vi "Mes配置.vi"() -> (1 "MES[]":T1(array[cluster]), 3 "MES 配置 2":T2={"SITE"="A157", "OPERATION"="Z-TEST", "QTY"="1", "ACTIVITY"="", "RESOURCE"="A-6-Z-TEST", "NC_CODE"="Z-TEST_FAIL", "IP"="10.9.30.175", "PORT"="50100", "URL"="/manufacturing/IntegrationServlet?InterType=XML&message="})   [LabVIEW 2011]
uses:
  Button.ctl
panel:
  in  "MES 配置":T2={"SITE"="A157", "OPERATION"="Z-TEST", "QTY"="1", "ACTIVITY"="", "RESOURCE"="A-6-Z-TEST", "NC_CODE"="Z-TEST_FAIL", "IP"="10.9.30.175", "PORT"="50100", "URL"="/manufacturing/IntegrationServlet?InterType=XML&message="}
  in  "delete":T3
  in  "input":T3
  in  "新建":T3
  in  "Exit":T3
  in  "所有MES配置表":i32(listbox)
  in  "MES配置信息名称":string
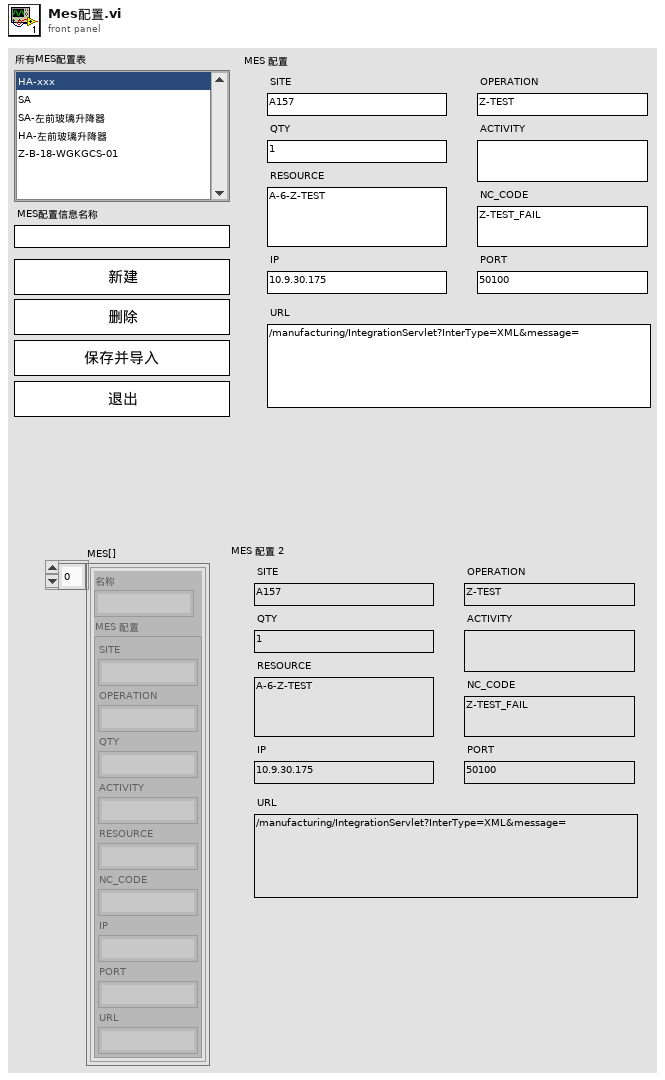
[diagram p1: front panel]
types:
  T1 = cluster{"名称":string, "MES 配置":cluster{"SITE":string, "OPERATION":string, "QTY":string, "ACTIVITY":string, "RESOURCE":string, "NC_CODE":string, "IP":string, "PORT":string, "URL":string}}[]
  T2 = cluster{"SITE":string, "OPERATION":string, "QTY":string, "ACTIVITY":string, "RESOURCE":string, "NC_CODE":string, "IP":string, "PORT":string, "URL":string}
  T3 = typedef "Button.ctl" = bool
  T4 = cluster{"名称":string, "电机位置":cluster{"左工位工作位置":cluster{"Axis":i16, "Distance":i32, "StrVel":i32, "MaxVel":i32}, "左工位抬起开关位置":cluster{"Axis":i16, "Distance":i32, "StrVel":i32, "MaxVel":i32}, "左工位按下开关位置":cluster{"Axis":i16, "Distance":i32, "StrVel":i32, "MaxVel":i32}, "右工位工作位置":cluster{"Axis":i16, "Distance":i32, "StrVel":i32, "MaxVel":i32}, "右工位抬起开关位置":cluster{"Axis":i16, "Distance":i32, "StrVel":i32, "MaxVel":i32}, "右工位按下开关位置":cluster{"Axis":i16, "Distance":i32, "StrVel":i32, "MaxVel":i32}}}
  T5 = cluster{"名称":string, "判定条件":cluster{"A1-A2电阻":cluster{"上限":dbl, "下限":dbl, "单位":string}, "A3-A4电阻":cluster{"上限":dbl, "下限":dbl, "单位":string}, "A4-A5电阻":cluster{"上限":dbl, "下限":dbl, "单位":string}, "A5-A6电阻":cluster{"上限":dbl, "下限":dbl, "单位":string}, "A1-A3电阻":cluster{"上限":dbl, "下限":dbl, "单位":string}, "A2-A6电阻":cluster{"上限":dbl, "下限":dbl, "单位":string}, "A1导地A3-A5电压":cluster{"上限":dbl, "下限":dbl, "单位":string}, "A2导地A6-A5电压":cluster{"上限":dbl, "下限":dbl, "单位":string}, "抬起开关A3-A5电压":cluster{"上限":dbl, "下限":dbl, "单位":string}, "按下开关A6-A5电压":cluster{"上限":dbl, "下限":dbl, "单位":string}, "背光电流":cluster{"上限":dbl, "下限":dbl, "单位":string}, "A1导地A6-A5电压":cluster{"上限":dbl, "下限":dbl, "单位":string}, "A2导地A3-A5电压":cluster{"上限":dbl, "下限":dbl, "单位":string}}}
  T6 = cluster{"名称":string, "MES 配置":cluster{"SITE":string, "OPERATION":string, "QTY":string, "ACTIVITY":string, "RESOURCE":string, "NC_CODE":string, "IP":string, "PORT":string, "URL":string}}
  T7 = enum16{"open", "replace", "create", "open or create", "replace or create", "replace or create with confirmation"}
  T8 = cluster{"SITE":string, "OPERATION":string, "QTY":string, "ACTIVITY":string, "RESOURCE":string, "NC_CODE":string, "IP":string, "PORT":string, "URL":string}[]
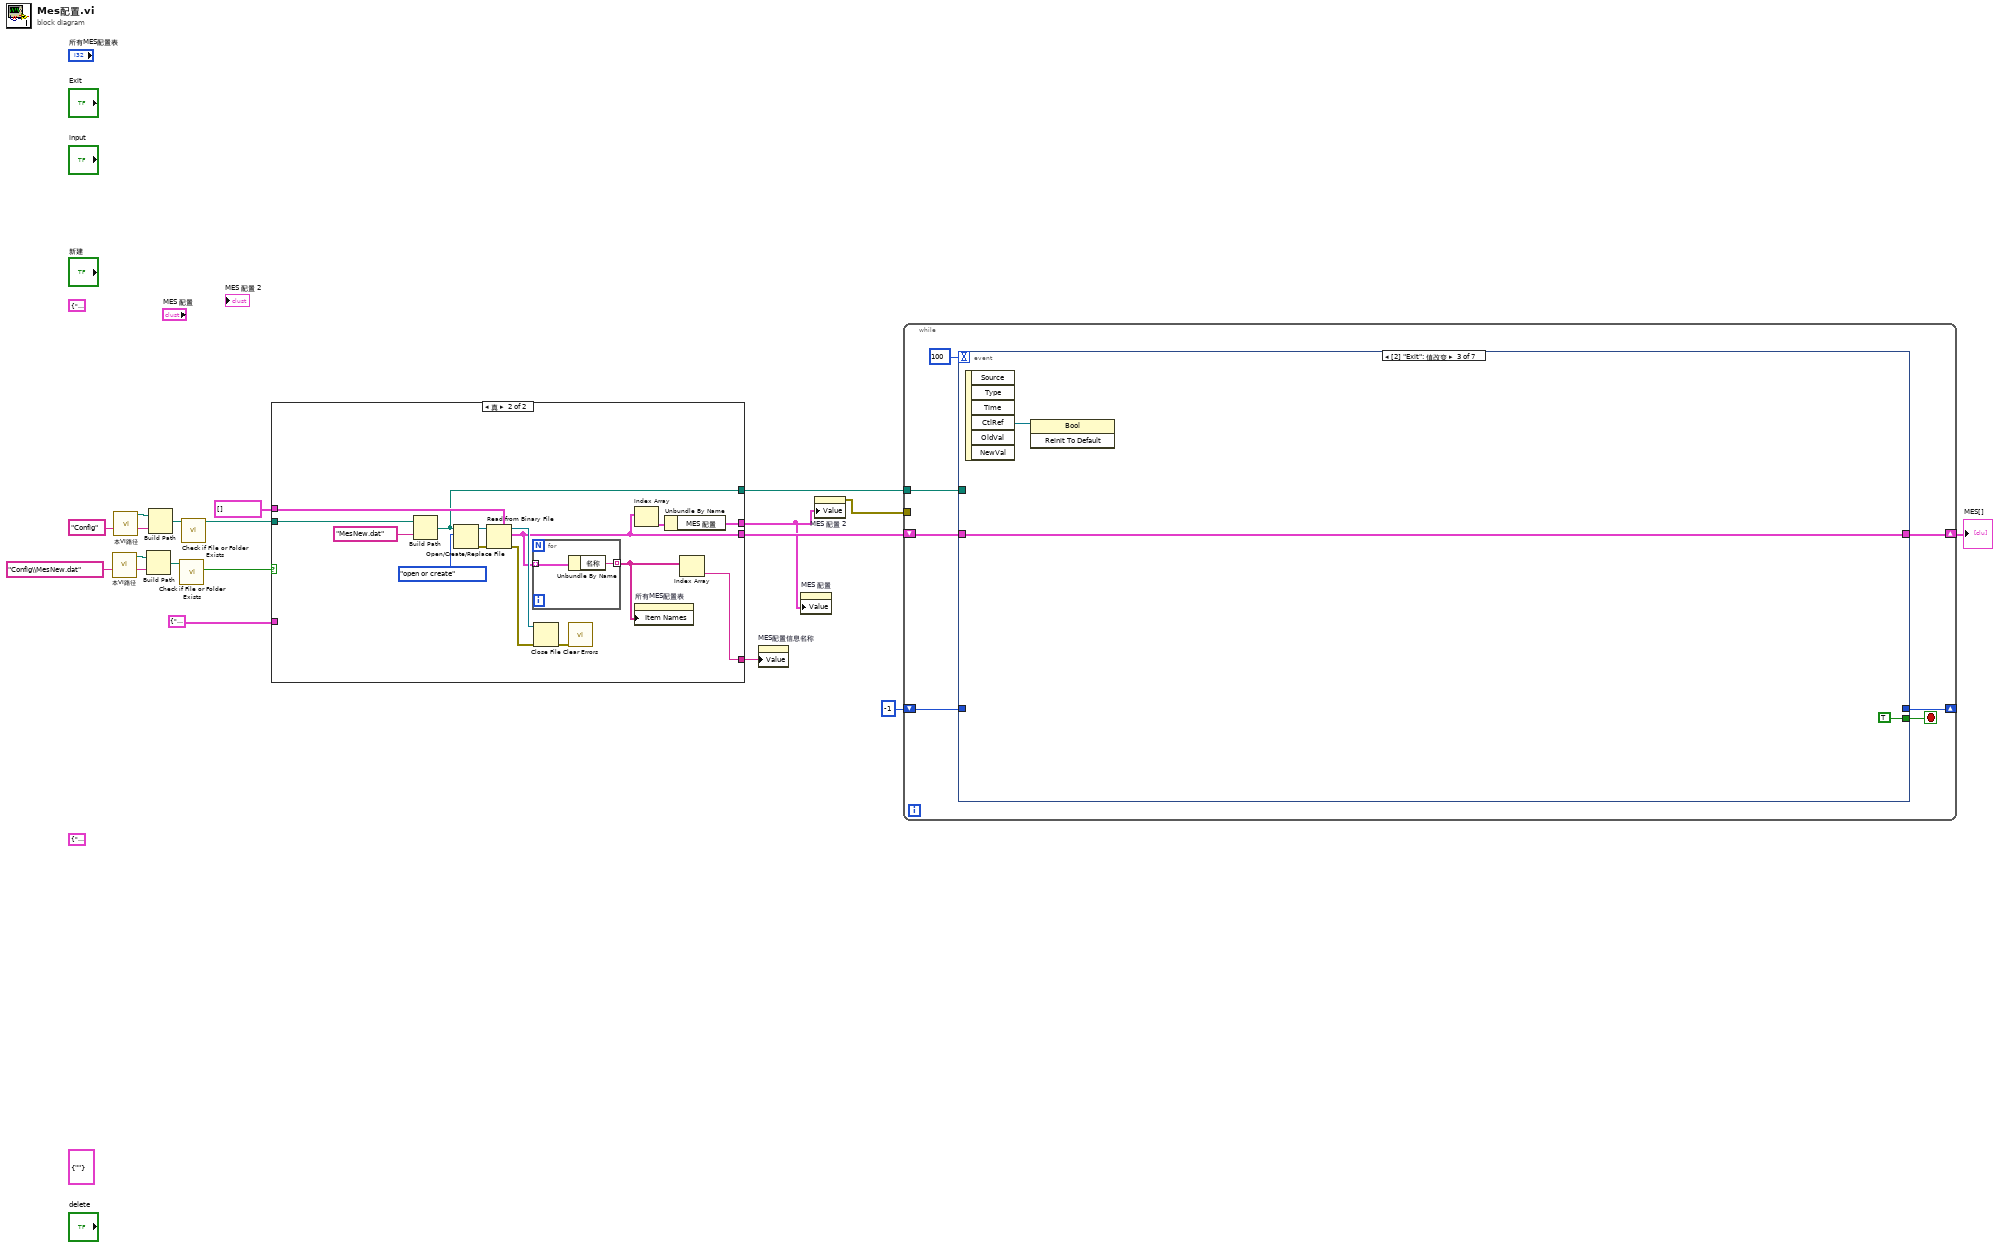
[diagram p0: block diagram]
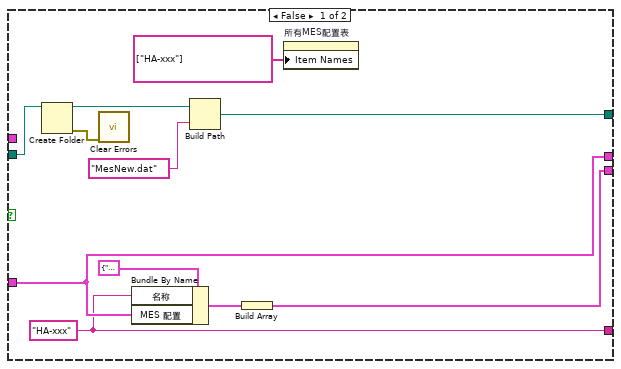
[diagram p2: hidden frame]
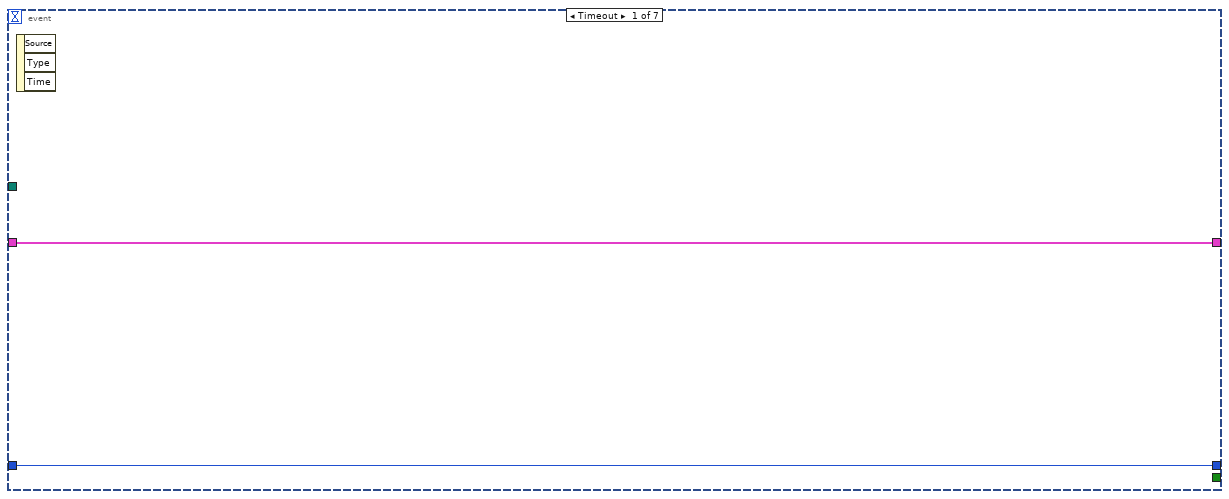
[diagram p3: hidden frame]
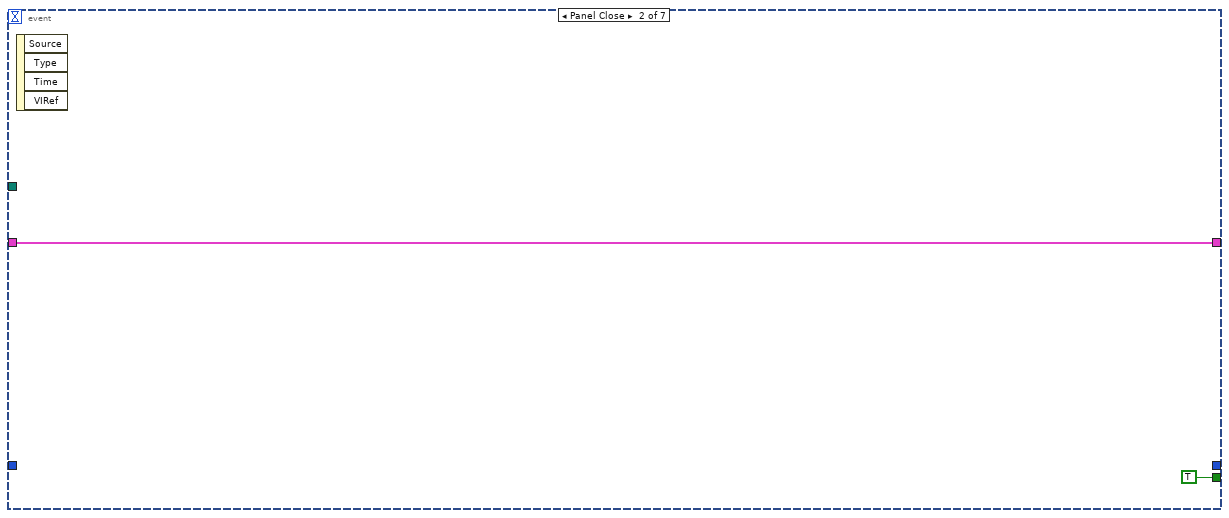
[diagram p4: hidden frame]
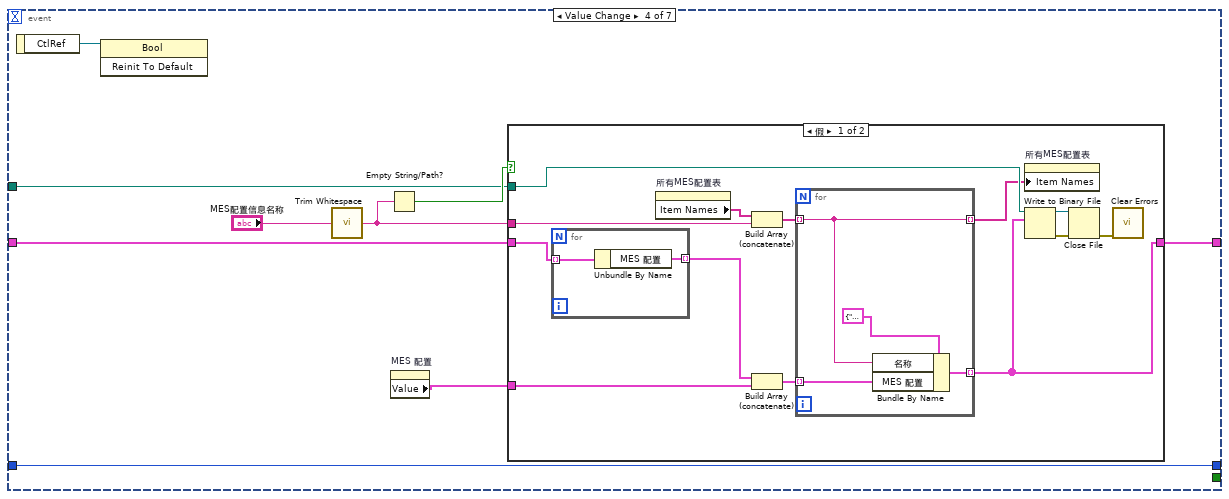
[diagram p5: hidden frame]
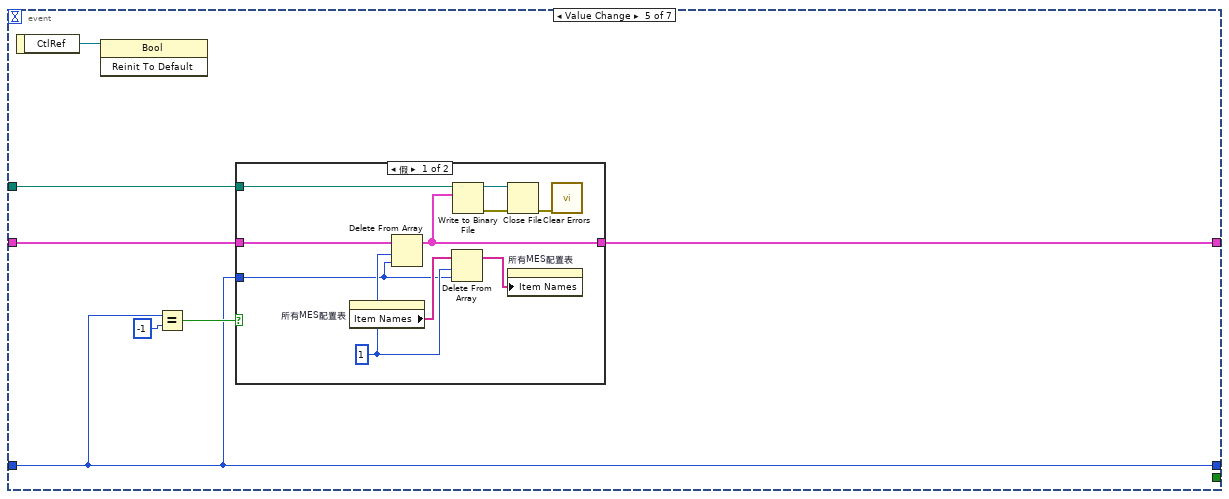
[diagram p7: hidden frame]
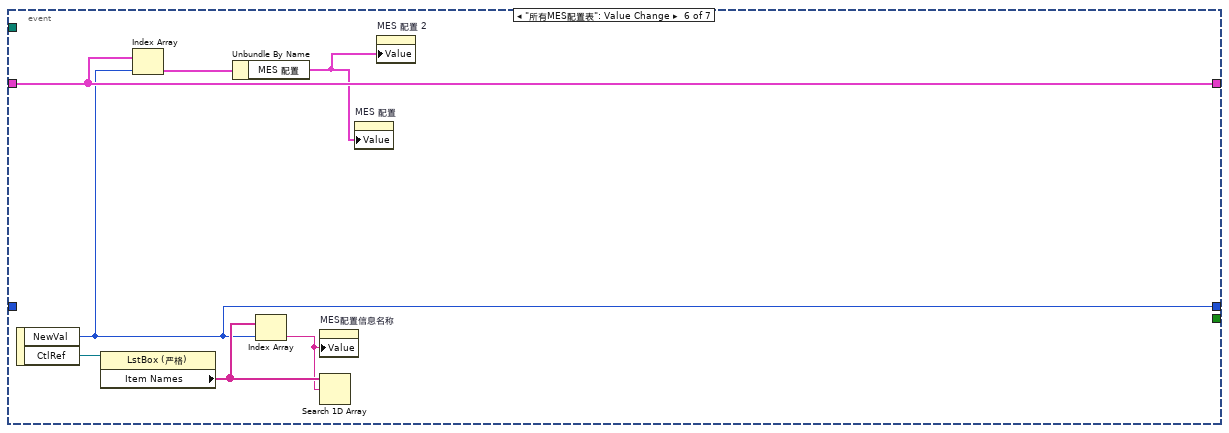
[diagram p9: hidden frame]
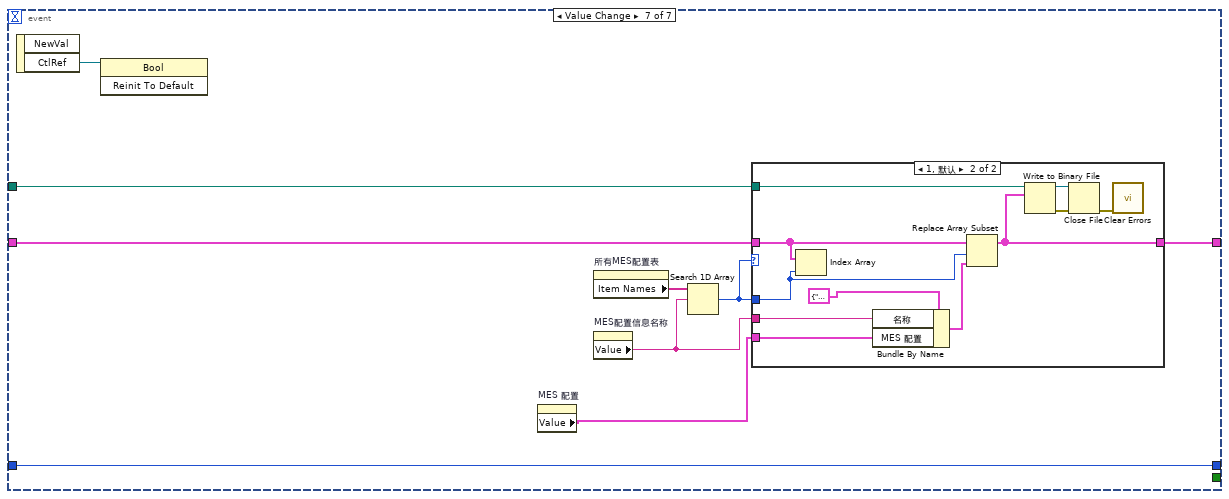
[diagram p10: hidden frame]
diagram:
  (unwired) T4 {"名称"="Config", "电机位置"={"左工位工作位置"={"Axis"=0, "Distance"=200, "StrVel"=500, "MaxVel"=3000}, "左工位抬起开关位置"={"Axis"=0, "Distance"=200, "StrVel"=500, "MaxVel"=3000}, "左工位按下开关位置"={"Axis"=0, "Distance"=200, "StrVel"=500, "MaxVel"=3000}, "右工位工作位置"={"Axis"=0, "Distance"=200, "StrVel"=500, "MaxVel"=3000}, "右工位抬起开关位置"={"Axis"=0, "Distance"=200, "StrVel"=500, "MaxVel"=3000}, "右工位按下开关位置"={"Axis"=0, "Distance"=200, "StrVel"=500, "MaxVel"=3000}}}
  (unwired) T5 {"名称"="", "判定条件"={"A1-A2电阻"={"上限"=390.0, "下限"=355.0, "单位"="Ω"}, "A3-A4电阻"={"上限"=-1.0, "下限"=-1.0, "单位"=""}, "A4-A5电阻"={"上限"=-1.0, "下限"=-1.0, "单位"="Ω"}, "A5-A6电阻"={"上限"=-1.0, "下限"=-1.0, "单位"="Ω"}, "A1-A3电阻"={"上限"=-1.0, "下限"=-1.0, "单位"="Ω"}, "A2-A6电阻"={"上限"=-1.0, "下限"=-1.0, "单位"="Ω"}, "A1导地A3-A5电压"={"上限"=14.05, "下限"=13.95, "单位"="V"}, "A2导地A6-A5电压"={"上限"=0.0, "下限"=0.0, "单位"="V"}, "抬起开关A3-A5电压"={"上限"=0.0, "下限"=0.0, "单位"="V"}, "按下开关A6-A5电压"={"上限"=0.0, "下限"=0.0, "单位"="V"}, "背光电流"={"上限"=35.0, "下限"=25.0, "单位"="mA"}, "A1导地A6-A5电压"={"上限"=14.05, "下限"=13.95, "单位"="V"}, "A2导地A3-A5电压"={"上限"=0.0, "下限"=0.0, "单位"="V"}}}
  (unwired) cluster{"名称":string} {"名称"=""}
  n1 = call "本VI路径.vi"() -> ("stripped path"=w5:path)  [unwired: 11 in]
  n2 = call "本VI路径.vi"() -> ("stripped path"=w10:path)  [unwired: 11 in]
  n3 = Build Path(base path=w5, name or relative path="Config\\MesNew.dat" ("名称或相对路径")) -> (appended path=w3:path)
  n4 = Build Path(base path=w10, name or relative path="Config" ("名称或相对路径")) -> (appended path=w17:path)
  n5 = call <vilib>:"Check if File or Folder Exists.vi"("path"=w3) -> ("file or folder exists?"=w2:bool)  [unwired: 8 in, 2 out]
  n6 = call <vilib>:"Check if File or Folder Exists.vi"("path"=w17) -> ("dup path"=w15:path)  [unwired: 8 in, 2 out]
  n7 = case shown="真" w2 {
    tunnel: w15 -> [w22 w36]
    tunnel: T1 [] -> [_ w41]
    tunnel: [w20 w39] -> w6
    tunnel: T2 {"SITE"="A157", "OPERATION"="Z-TEST", "QTY"="1", "ACTIVITY"="", "RESOURCE"="A-6-Z-TEST", "NC_CODE"="Z-TEST_FAIL", "IP"="10.9.30.175", "PORT"="50100", "URL"="/manufacturing/IntegrationServlet?InterType=XML&message="} ("MES 配置 2") -> [w20 _]
    tunnel: [w26 w38] -> w13
    tunnel: [w18 w35] -> w12
    tunnel: [w19 w30] -> w9
    frame False {
      w19 = "HA-xxx"
      n8 = Create Folder(path (use dialog)=w22) -> (created path=w23:path, error out=w25:errorcluster)  [unwired: 2 in, 1 out]
      n9 = call <vilib>:"Clear Errors.vi"("error in (no error)"=w25) -> ()  [unwired: 6 in, 1 out]
      n10 = Bundle By Name(cluster=T6 {"名称"="Config", "MES 配置"={"SITE"="A157", "OPERATION"="Z-TEST", "QTY"="1", "ACTIVITY"="", "RESOURCE"="A-6-Z-TEST", "NC_CODE"="Z-TEST_FAIL", "IP"="10.9.30.175", "PORT"="50100", "URL"="/manufacturing/IntegrationServlet?InterType=XML&message="}}, "名称"=w19, "MES 配置"=w20) -> (w27:T6)
      n11 = Build Path(base path=w23, name or relative path="MesNew.dat" ("名称或相对路径")) -> (appended path=w18:path)
      n12 = Build Array(w27) -> (w26:T1)
      n13 = property on="所有MES配置表" class="LstBox (严格)"("Item Names"=string[] ["HA-xxx"] ("项名")) -> ()  [unwired: 2 in, 2 out]
    }
    frame True {
      n14 = Build Path(base path=w36, name or relative path="MesNew.dat" ("名称或相对路径")) -> (appended path=w35:path)
      n15 = Open/Create/Replace File(file path (use dialog)=w35, operation (0:open)=T7."open or create" ("操作(0:open)")) -> (refnum out=w33:refnum<file>, error out=w29:errorcluster)  [unwired: 4 in, 1 out]
      n16 = Read from Binary File(5:w41, 8:w29, 11:w33) -> (0:w42:errorcluster, 2:w38:T1, 3:w43:refnum<file>)  [unwired: 3 in, 1 out]
      n17 = for {
        tunnel: w38 -> [w45] mode=indexing
        tunnel: [w44] -> w31 mode=indexing
        n18 = Unbundle By Name(w45) -> ("名称"=w44:string)
      }
      n19 = Close File(refnum=w43, error in=w42) -> (error out=w37:errorcluster)  [unwired: 1 out]
      n20 = call <vilib>:"Clear Errors.vi"("error in (no error)"=w37) -> ()  [unwired: 6 in, 1 out]
      n21 = Index Array(array=w38) -> (element=w40:T6)  [unwired: 1 in]
      n22 = property on="所有MES配置表" class="LstBox (严格)"("Item Names"=w31) -> ()  [unwired: 2 in, 2 out]
      n23 = Unbundle By Name(w40) -> ("MES 配置"=w39:T2)
      n24 = Index Array(array=w31) -> (element=w30:string)  [unwired: 1 in]
    }
  }
  n25 = property on="MES配置信息名称" class="Str"("Value"=w9) -> ()  [unwired: 2 in, 2 out]
  n26 = property on="MES 配置" class="Clust (严格)"("Value"=w6) -> ()  [unwired: 2 in, 2 out]
  n27 = property on="MES 配置 2" class="Clust (严格)"("Value"=w6) -> (error out=w7:errorcluster)  [unwired: 2 in, 1 out]
  n28 = while {
    tunnel: w7 -> [_]
    tunnel: w12 -> [w49]
    shift-right: [w48] -> w1
    shift-left: w13 -> [w50]
    shift-right: [w47] -> _
    shift-left: -1 ("NewVal") -> [w46]
    stop <- w51 stop-if-true
    n29 = event shown="[2] \"Exit\": 值改变" {
      selector: _ -> [_ _ _ _ _ _ _]
      dyn-events: _ -> [_ _ _ _ _ _ _]
      timeout: 100 -> [_ _ _ _ _ _ _]
      tunnel: [_ TRUE TRUE _ _ _ _] -> w51
      tunnel: w50 -> [w54 w56 w57 w64 w94 w111 w119]
      tunnel: w49 -> [_ _ _ w63 w93 _ w115]
      tunnel: [w54 w56 w57 w62 w92 w111 w117] -> w48
      tunnel: [w53 _ _ w61 w89 w110 w122] -> w47
      tunnel: w46 -> [w53 _ _ w61 w89 _ w122]
      event Timeout {
        n30 = event-data() -> ()  [unwired: 1 in, 3 out]
      }
      event Panel Close {
        n31 = event-data() -> ()  [unwired: 1 in, 4 out]
      }
      event Value Change {
        n32 = event-data() -> ("CtlRef"=w58:refnum<vi>)  [unwired: 1 in, 5 out]
        n33 = invoke class="Bool" method="Reinit To Default"(reference=w58) -> ()  [unwired: 2 in, 3 out]
      }
      event Value Change {
        n34 = event-data() -> ("CtlRef"=w68:refnum<vi>)  [unwired: 1 in]
        n35 = invoke class="Bool" method="Reinit To Default"(reference=w68) -> ()  [unwired: 2 in, 3 out]
        n36 = call <vilib>:"Trim Whitespace.vi"("string"="MES配置信息名称") -> ("trimmed string"=w65:string)  [unwired: 1 in]
        n37 = Empty String/Path?(string/path=w65) -> (empty?=w66:bool)
        n38 = property on="MES 配置" class="Clust (严格)"() -> ("Value"=w60:T2)  [unwired: 2 in, 2 out]
        n39 = case shown="假" w66 {
          tunnel: w65 -> [w80 _]
          tunnel: w64 -> [w79 w88]
          tunnel: w60 -> [w69 _]
          tunnel: w63 -> [w75 _]
          tunnel: [w71 w88] -> w62
          frame False {
            n40 = for {
              tunnel: w79 -> [w87] mode=indexing
              tunnel: [w86] -> w78 mode=indexing
              n41 = Unbundle By Name(w87) -> ("MES 配置"=w86:T2)
            }
            n42 = property on="所有MES配置表" class="LstBox (严格)"() -> ("Item Names"=w81:string[])  [unwired: 2 in, 2 out]
            n43 = Build Array (concatenate)(w81, w80) -> (w77:string[])
            n44 = Build Array (concatenate)(w78, w69) -> (w76:T8)
            n45 = for {
              tunnel: w77 -> [w83] mode=indexing
              tunnel: w76 -> [w85] mode=indexing
              tunnel: [w84] -> w71 mode=indexing
              tunnel: [w83] -> w70 mode=indexing
              n46 = Bundle By Name(cluster=T6 {"名称"="Config", "MES 配置"={"SITE"="A157", "OPERATION"="Z-TEST", "QTY"="1", "ACTIVITY"="", "RESOURCE"="A-6-Z-TEST", "NC_CODE"="Z-TEST_FAIL", "IP"="10.9.30.175", "PORT"="50100", "URL"="/manufacturing/IntegrationServlet?InterType=XML&message="}}, "名称"=w83, "MES 配置"=w85) -> (w84:T6)
            }
            n47 = property on="所有MES配置表" class="LstBox (严格)"("Item Names"=w70) -> ()  [unwired: 2 in, 2 out]
            n48 = Write to Binary File(file (use dialog)=w75, data=w71) -> (refnum out=w74:refnum<file>, error out=w73:errorcluster)  [unwired: 4 in, 1 out]
            n49 = Close File(refnum=w74, error in=w73) -> (error out=w72:errorcluster)  [unwired: 1 out]
            n50 = call <vilib>:"Clear Errors.vi"("error in (no error)"=w72) -> ()  [unwired: 6 in, 1 out]
          }
          frame True {
          }
        }
      }
      event Value Change {
        n51 = event-data() -> ("CtlRef"=w95:refnum<vi>)  [unwired: 1 in]
        n52 = invoke class="Bool" method="Reinit To Default"(reference=w95) -> ()  [unwired: 2 in, 3 out]
        n53 = Equal?(x=w89, y=-1) -> (x = y?=w91:bool)
        n54 = case shown="假" w91 {
          tunnel: w94 -> [w99 w106]
          tunnel: w93 -> [w105 _]
          tunnel: [w97 w106] -> w92
          tunnel: w89 -> [w98 _]
          frame False {
            w100 = 1 ("长度")
            n55 = property on="所有MES配置表" class="LstBox (严格)"() -> ("Item Names"=w101:string[])  [unwired: 2 in, 2 out]
            n56 = Delete From Array(array=w99, length=w100, index=w98) -> (array with subset deleted=w97:T1)  [unwired: 1 out]
            n57 = Delete From Array(array=w101, length=w100, index=w98) -> (array with subset deleted=w96:string[])  [unwired: 1 out]
            n58 = Write to Binary File(file (use dialog)=w105, data=w97) -> (refnum out=w104:refnum<file>, error out=w103:errorcluster)  [unwired: 4 in, 1 out]
            n59 = Close File(refnum=w104, error in=w103) -> (error out=w102:errorcluster)  [unwired: 1 out]
            n60 = property on="所有MES配置表" class="LstBox (严格)"("Item Names"=w96) -> ()  [unwired: 2 in, 2 out]
            n61 = call <vilib>:"Clear Errors.vi"("error in (no error)"=w102) -> ()  [unwired: 6 in, 1 out]
          }
          frame True {
          }
        }
      }
      event "所有MES配置表": Value Change {
        n62 = event-data() -> ("NewVal"=w110:i32, "CtlRef"=w113:refnum<vi>)  [unwired: 1 in]
        n63 = property class="LstBox (严格)"(reference=w113) -> ("Item Names"=w112:string[])  [unwired: 1 in, 2 out]
        n64 = Index Array(array=w111, index=w110) -> (element=w109:T6)
        n65 = Unbundle By Name(w109) -> ("MES 配置"=w107:T2)
        n66 = Index Array(array=w112, index=w110) -> (element=w108:string)
        n67 = property on="MES配置信息名称" class="Str"("Value"=w108) -> ()  [unwired: 2 in, 2 out]
        n68 = Search 1D Array(1D array=w112, element=w108) -> ()  [unwired: 1 in, 1 out]
        n69 = property on="MES 配置" class="Clust (严格)"("Value"=w107) -> ()  [unwired: 2 in, 2 out]
        n70 = property on="MES 配置 2" class="Clust (严格)"("Value"=w107) -> ()  [unwired: 2 in, 2 out]
      }
      event Value Change {
        n71 = event-data() -> ("CtlRef"=w121:refnum<vi>)  [unwired: 1 in, 1 out]
        n72 = invoke class="Bool" method="Reinit To Default"(reference=w121) -> ()  [unwired: 2 in, 3 out]
        n73 = property on="MES 配置" class="Clust (严格)"() -> ("Value"=w114:T2)  [unwired: 2 in, 2 out]
        n74 = property on="所有MES配置表" class="LstBox (严格)"() -> ("Item Names"=w120:string[])  [unwired: 2 in, 2 out]
        n75 = property on="MES配置信息名称" class="Str"() -> ("Value"=w116:string)  [unwired: 2 in, 2 out]
        n76 = Search 1D Array(1D array=w120, element=w116) -> (index of element=w118:i32)  [unwired: 1 in]
        n77 = case shown="1, 默认" w118 {
          tunnel: w119 -> [w123 w134]
          tunnel: w118 -> [_ w133]
          tunnel: [w123 w126] -> w117
          tunnel: w114 -> [_ w132]
          tunnel: w116 -> [_ w131]
          tunnel: w115 -> [_ w125]
          frame -1 {
          }
          frame 1, Default {
            n78 = Index Array(array=w134, index=w133) -> ()  [unwired: 1 out]
            n79 = Bundle By Name(cluster=T6 {"名称"="Config", "MES 配置"={"SITE"="A157", "OPERATION"="Z-TEST", "QTY"="1", "ACTIVITY"="", "RESOURCE"="A-6-Z-TEST", "NC_CODE"="Z-TEST_FAIL", "IP"="10.9.30.175", "PORT"="50100", "URL"="/manufacturing/IntegrationServlet?InterType=XML&message="}}, "名称"=w131, "MES 配置"=w132) -> (w130:T6)
            n80 = Replace Array Subset(array=w134, new element=w130, index=w133) -> (w126:T1)
            n81 = Write to Binary File(file (use dialog)=w125, data=w126) -> (refnum out=w129:refnum<file>, error out=w128:errorcluster)  [unwired: 4 in, 1 out]
            n82 = Close File(refnum=w129, error in=w128) -> (error out=w127:errorcluster)  [unwired: 1 out]
            n83 = call <vilib>:"Clear Errors.vi"("error in (no error)"=w127) -> ()  [unwired: 6 in, 1 out]
          }
        }
      }
    }
  }
  "MES[]" <- w1
